vi "WaitforTelapsed.vi"(0 "exp time in mu sec":u32) -> ()   [LabVIEW 2014]
uses:
  ESLSCDLL.dll
panel:
  out "too short":bool
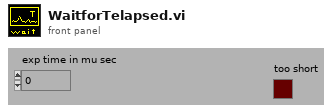
[diagram p1: front panel]
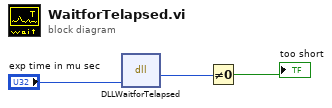
[diagram p0: block diagram]
diagram:
  n1 = dll-call lib="C:/Users/Gerhard/Documents/New64/lv/1cam/board.vis/ESLSCDLL.dll" fn="DLLWaitforTelapsed"("musec"="exp time in mu sec") -> ("Rückgabetyp"=w2:u8)  [unwired: 4 in, 2 out]
  n2 = Not Equal To 0?(x=w2) -> (x != 0?=→"too short":bool)
